vi "KRH Duel Controller Solenoid.vi"(8 "Joystick 1 Input":T1, 10 "Joystick Select":bool, 11 "Joystick 0 Input":T1) -> (2 "Solenoid Output":T1)   [LabVIEW 2015]
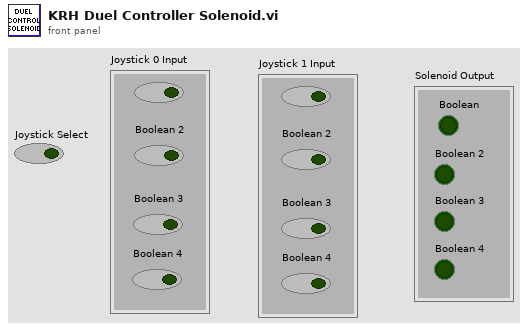
[diagram p1: front panel]
types:
  T1 = cluster{"Boolean":bool, "Boolean 2":bool, "Boolean 3":bool, "Boolean 4":bool}
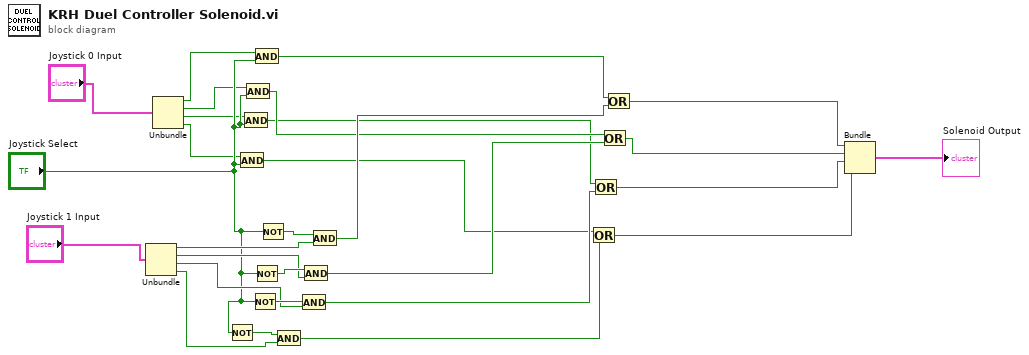
[diagram p0: block diagram]
diagram:
  n1 = Unbundle("Joystick 1 Input") -> ("Boolean"=w14:bool, "Boolean 2"=w13:bool, "Boolean 3"=w12:bool, "Boolean 4"=w11:bool)
  n2 = Unbundle("Joystick 0 Input") -> ("Boolean"=w9:bool, "Boolean 2"=w8:bool, "Boolean 3"=w7:bool, "Boolean 4"=w6:bool)
  n3 = Not(x="Joystick Select") -> (.not. x?=w18:bool)
  n4 = And(x=w6, y="Joystick Select") -> (x .and. y?=w20:bool)
  n5 = And(x=w7, y="Joystick Select") -> (x .and. y?=w22:bool)
  n6 = And(x=w8, y="Joystick Select") -> (x .and. y?=w24:bool)
  n7 = Not(x="Joystick Select") -> (.not. x?=w17:bool)
  n8 = And(x=w9, y="Joystick Select") -> (x .and. y?=w25:bool)
  n9 = Not(x="Joystick Select") -> (.not. x?=w16:bool)
  n10 = Not(x="Joystick Select") -> (.not. x?=w15:bool)
  n11 = And(x=w18, y=w11) -> (x .and. y?=w19:bool)
  n12 = And(x=w17, y=w12) -> (x .and. y?=w21:bool)
  n13 = And(x=w16, y=w13) -> (x .and. y?=w23:bool)
  n14 = And(x=w15, y=w14) -> (x .and. y?=w26:bool)
  n15 = Or(x=w20, y=w19) -> (x .or. y?=w2:bool)
  n16 = Or(x=w22, y=w21) -> (x .or. y?=w3:bool)
  n17 = Or(x=w24, y=w23) -> (x .or. y?=w4:bool)
  n18 = Or(x=w25, y=w26) -> (x .or. y?=w5:bool)
  n19 = Bundle(w5, w4, w3, w2) -> (→"Solenoid Output":cluster{bool, bool, bool, bool})  [unwired: 1 in]
